vi "LawOfSines.vi"(1 "Opposite Unknown Angle":dbl, 2 "Opposite Known Angle":dbl, 3 "Known Angle":dbl) -> (0 "Unknown Angle":dbl)   [LabVIEW 2016]
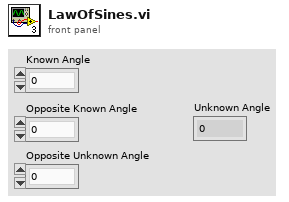
[diagram p1: front panel]
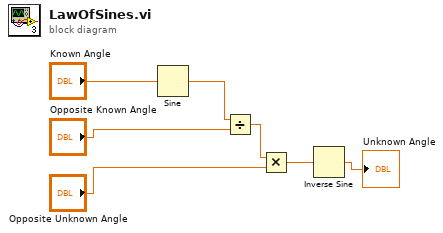
[diagram p0: block diagram]
diagram:
  n1 = Sine(x="Known Angle") -> (sin(x)=w6:dbl)
  n2 = Divide(x=w6, y="Opposite Known Angle") -> (x/y=w3:dbl)
  n3 = Multiply(x=w3, y="Opposite Unknown Angle") -> (x*y=w1:dbl)
  n4 = Inverse Sine(1:w1) -> (0:→"Unknown Angle":dbl)
